vi "PT3_Read.vi"(7 "Start From Top":bool, 8 "error in":errorcluster, 10 "Data count":i32=1, 11 "refnum in":refnum<file>) -> (0 "error out":errorcluster, 2 "Data out":u32[](array[numeric]), 3 "refnum out":refnum<file>, 4 "EOF?":bool)   [LabVIEW 8.6]
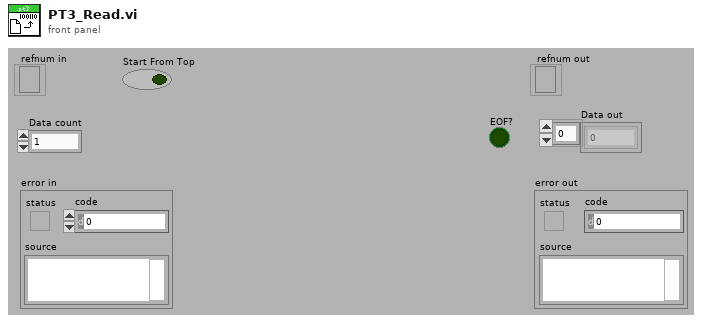
[diagram p1: front panel]
types:
  T1 = enum16{"big-endian, network order", "native, host order", "little-endian"}
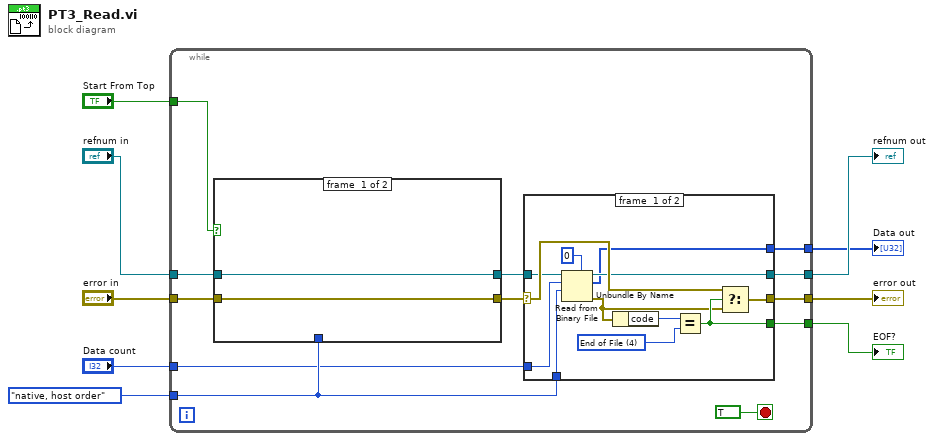
[diagram p0: block diagram]
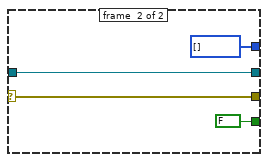
[diagram p2: hidden frame]
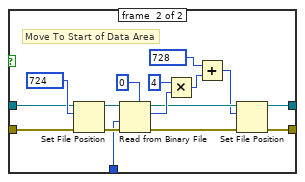
[diagram p3: hidden frame]
diagram:
  n1 = while {
    tunnel: "error in" -> [w20]
    tunnel: "refnum in" -> [w19]
    tunnel: T1."native, host order" ("byte order (0:big-endian, network order)") -> [w17]
    tunnel: "Start From Top" -> [w18]
    tunnel: [w15] -> w5
    tunnel: [w14] -> w4
    tunnel: "Data count" -> [w12]
    tunnel: [w11] -> w2
    tunnel: [w10] -> w1
    stop <- TRUE stop-if-true
    n2 = case shown="True" w18 {
      tunnel: w20 -> [w39 w54]
      tunnel: w19 -> [w38 w53]
      tunnel: w17 -> [_ w49]
      tunnel: [w39 w41] -> w16
      tunnel: [w38 w40] -> w13
      frame #0 {
      }
      frame #1 {
        # "Move To Start of Data Area"
        n3 = Set File Position(offset (in bytes) (0)=i64 724, refnum=w53, error in=w54) -> (refnum out=w50:refnum<file>, error out=w51:errorcluster)  [unwired: 1 out]
        n4 = Read from Binary File(5:0, 8:w51, 9:w49, 11:w50) -> (0:w44:errorcluster, 2:w48:i32, 3:w43:refnum<file>)  [unwired: 3 out]
        n5 = Multiply(x=4, y=w48) -> (x*y=w46:i32)
        n6 = Add(x=i64 728 ("offset (in bytes) (0)"), y=w46) -> (x+y=w42:i64)
        n7 = Set File Position(offset (in bytes) (0)=w42, refnum=w43, error in=w44) -> (refnum out=w40:refnum<file>, error out=w41:errorcluster)  [unwired: 1 out]
      }
    }
    n8 = case shown="No Error" w16 {
      selector: w16 -> [w28 w37]
      tunnel: w17 -> [w33 _]
      tunnel: [w26 w37] -> w14
      tunnel: [w29 FALSE] -> w15
      tunnel: w13 -> [w25 w35]
      tunnel: [w24 w35] -> w11
      tunnel: w12 -> [w23 _]
      tunnel: [w22 u32[] []] -> w10
      frame #0 {
        w31 = 4 items=["No Error", "Manager Argument Error", "Memory Full", "Out of Zone", "End of File", "File Already Open", "Generic File IO Error", "File Not Found", "File Permission Error", "Disk Full", "Duplicate Path", "Too Many Files Open", "Not Enabled", "Resource File Not Found", "Cannot Add Resource", "Resource Not Found", "Image Not Found", "Image Memory Error", "Pen Does Not Exist", "Config Bad Type", "Config Token Not Found", "Config Parse Error", "Config Memory Error", "Bad External Code Format", "Bad External Code Offset", "External Code Not Present", "Null Window", "Destroy Window Mixup", "Null Menu", "Print Aborted", "Bad Print Record", "Print Driver Error", "Windows Error During Print", "Memory Error During Print", "Print Dialog Error", "Generic Print Error", "Invalid Device Refnum", "Device Not Found", "Device Parameter Error", "Device Unit Error", "Can't Open Device", "Device Call Aborted", "Generic Error", "Cancelled By User", "Object ID Too Low", "Object ID Too High", "Object Not In Heap", "Unknown Heap", "Bad DefProc ID", "DefProc Not In Table", "Message Out Of Range", "Null Method", "Unknown Message", "Manager Call Not Supported"]
        n9 = Read from Binary File(5:u32 0, 9:w33, 10:w23, 11:w25) -> (0:w27:errorcluster, 2:w22:u32[], 3:w24:refnum<file>)  [unwired: 1 in, 2 out]
        n10 = Unbundle By Name(w27) -> ("code"=w30:i32)
        n11 = Equal?(x=w30, y=w31) -> (x = y?=w29:bool)
        n12 = Select(t=w28, s=w29, f=w27) -> (s? t:f=w26:errorcluster)
      }
      frame #1 {
      }
    }
  }
  "refnum out" <- w2
  "error out" <- w4
  "EOF?" <- w5
  "Data out" <- w1
